vi "Neg Binomial Moments.vi"(9 "p":dbl=0.5, 10 "x":dbl=5.0) -> (0 "error":i32, 2 "variance":dbl=10.0, 3 "mean":dbl=5.0)   [LabVIEW 2020, in "NI_Gmath.lvlib"]
doc: "Returns the expected mean and variance of the random variate X, where X describes the selected distribution type. You must manually select the polymorphic instance to use."
uses:
  NI_Gmath.lvlib
  st_error_code.ctl
panel:
  # "Neg Binomial Moments"
  # "successes"
  # "probability"
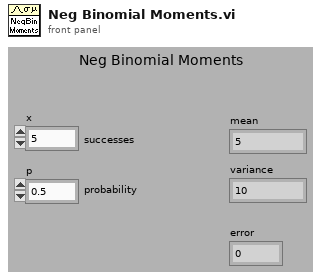
[diagram p1: front panel]
types:
  T1 = typedef "NI_Gmath.lvlib/st_error_code.ctl" = i32
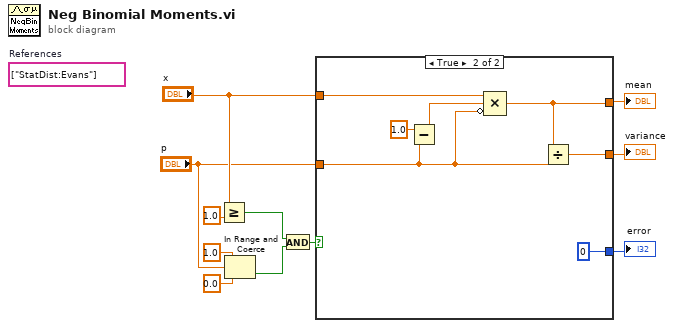
[diagram p0: block diagram]
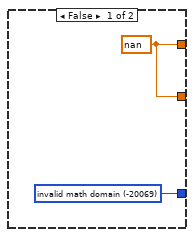
[diagram p2: hidden frame]
diagram:
  (unwired) string[] ["StatDist:Evans"]  # References
  n1 = Greater Or Equal?(x="x", y=1.0) -> (x >= y?=w5:bool)
  n2 = In Range and Coerce(upper limit=1.0, x="p", lower limit=0.0) -> (In Range?=w1:bool)  [unwired: 1 out]
  n3 = And(x=w5, y=w1) -> (x .and. y?=w4:bool)
  n4 = case shown="True" w4 {
    tunnel: [w13 w16] -> w11
    tunnel: [w13 w14] -> w10
    tunnel: [w12 0 ("error")] -> w9
    tunnel: "x" -> [_ w18]
    tunnel: "p" -> [_ w15]
    frame False {
      w12 = T1 -20069 items=["invalid math domain"=-20069, "Fourier interpolation size m >= n"=-20070, "empty array"=-20003] ("stat interp error code")
      w13 = nan
    }
    frame True {
      n5 = Subtract(x=1.0, y=w15) -> (x-y=w17:dbl)
      n6 = Compound Arithmetic op=MULTIPLY(w18, w17, invert w15) -> (w16:dbl)
      n7 = Divide(x=w16, y=w15) -> (x/y=w14:dbl)
    }
  }
  "error" <- w9
  "mean" <- w11
  "variance" <- w10
